vi "Config Limit Setting.vi"(0 "VISA resource name":refnum<visa-resource-name>, 5 "Source Setting (T:Voltage)":bool=TRUE, 7 "High Limit (1.00E+3)":dbl=1000.0 format="%^.2e", 11 "error in (no error)":errorcluster) -> (4 "VISA resource name out":refnum<visa-resource-name>, 15 "error out":errorcluster)   [LabVIEW 2011, in "Stanford Research PS300 Series.lvlib"]
doc: "This VI configures the output source and then specifies the highest output value for that source."
uses:
  <instrlib>/Stanford Research PS300 Series/Stanford Research PS300 Series.lvlib
panel:
  # "Voltage\nCurrent"
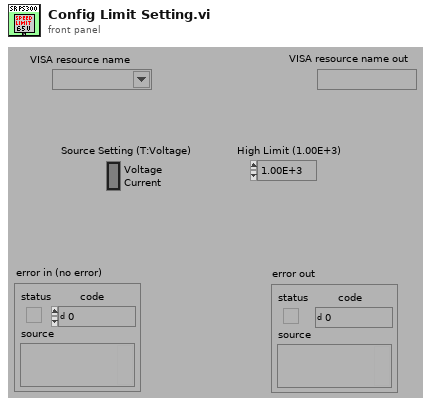
[diagram p1: front panel]
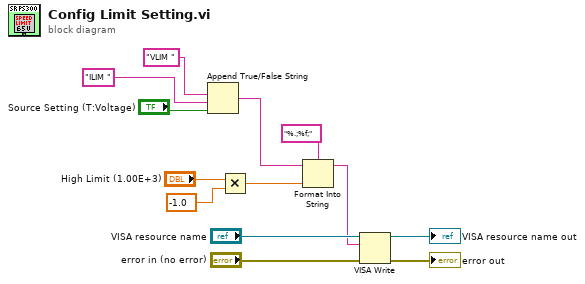
[diagram p0: block diagram]
diagram:
  n1 = Append True/False String(1:"Source Setting (T:Voltage)", 2:"ILIM " ("false string"), 3:"VLIM " ("true string")) -> (0:w8:string)  [unwired: 1 in]
  n2 = Multiply(x="High Limit (1.00E+3)", y=-1.0) -> (x*y=w1:dbl)
  n3 = Format Into String(format string="%.;%f;", initial string=w8, w1) -> (resulting string=w7:string)  [unwired: 1 in, 1 out]
  n4 = VISA Write(VISA resource name="VISA resource name", write buffer=w7, error in (no error)="error in (no error)") -> (VISA resource name out=→"VISA resource name out":refnum<visa-resource-name>, error out=→"error out":errorcluster)  [unwired: 1 out]
